vi "Tab as Wizard.vi"() -> ()   [LabVIEW 2014]
panel:
  in  "Next":bool
  in  "stop":bool
  in  "Tab Control":enum32{"Page 1", "Page 2", "Page 3", "Page 4"}(tab)
  # "Page 1"
  # "Page 2"
  # "Page 3"
  # "Page 4"
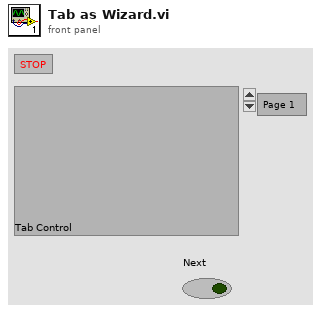
[diagram p1: front panel]
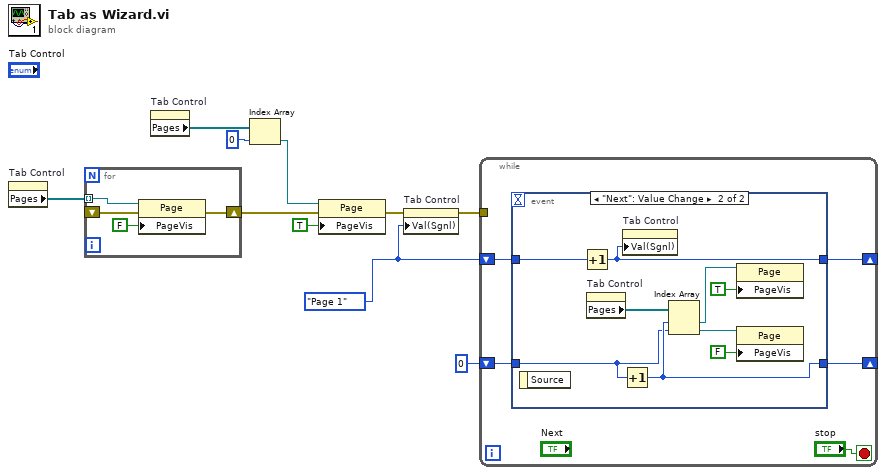
[diagram p0: block diagram]
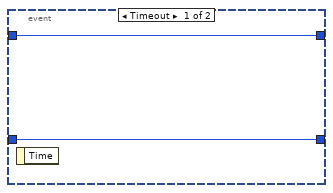
[diagram p2: hidden frame]
diagram:
  w1 = enum32{"Page 1", "Page 2", "Page 3", "Page 4"}."Page 1" ("Tab Control")
  n1 = property on="Tab Control" class="TabCtl (strict)"() -> ("Pages"=w8:refnum<vi>[])  [unwired: 2 in, 2 out]
  n2 = for {
    tunnel: w8 -> [w14] mode=indexing
    shift-right: [w12] -> w4
    shift-left: _ -> [w11]
    n3 = property class="Page"(reference=w14, error in=w11, "PageVis"=FALSE ("Page Visible")) -> (error out=w12:errorcluster)  [unwired: 1 out]
  }
  n4 = property on="Tab Control" class="TabCtl (strict)"() -> ("Pages"=w7:refnum<vi>[])  [unwired: 2 in, 2 out]
  n5 = Index Array(array=w7, index=0) -> (element=w5:refnum<vi>)
  n6 = property class="Page"(reference=w5, error in=w4, "PageVis"=TRUE ("Page Visible")) -> (error out=w2:errorcluster)  [unwired: 1 out]
  n7 = property on="Tab Control" class="TabCtl (strict)"(error in=w2, "Val(Sgnl)"=w1) -> (error out=w10:errorcluster)  [unwired: 1 in, 1 out]
  n8 = while {
    tunnel: w10 -> [_]
    shift-right: [w17] -> _
    shift-left: w1 -> [w18]
    shift-right: [w15] -> _
    shift-left: u16 0 -> [w16]
    stop <- "stop" stop-if-true
    n9 = event shown="[1] \"Next\": Value Change" {
      selector: _ -> [_ _]
      dyn-events: _ -> [_ _]
      timeout: _ -> [_ _]
      tunnel: w18 -> [w20 w30]
      tunnel: [w20 w29] -> w17
      tunnel: w16 -> [w21 w24]
      tunnel: [w21 w27] -> w15
      event Timeout {
        n10 = event-data() -> ()  [unwired: 1 in, 1 out]
      }
      event "Next": Value Change {
        n11 = event-data() -> ()  [unwired: 1 in, 1 out]
        n12 = Increment(x=w30) -> (x+1=w29:enum32{"Page 1", "Page 2", "Page 3", "Page 4"})
        n13 = property on="Tab Control" class="TabCtl (strict)"() -> ("Pages"=w28:refnum<vi>[])  [unwired: 2 in, 2 out]
        n14 = Increment(x=w24) -> (x+1=w27:u16)
        n15 = property on="Tab Control" class="TabCtl (strict)"("Val(Sgnl)"=w29) -> ()  [unwired: 2 in, 2 out]
        n16 = Index Array(array=w28, index #1=w27, index #2=w24) -> (element #1=w26:refnum<vi>, element #2=w23:refnum<vi>)
        n17 = property class="Page"(reference=w26, "PageVis"=TRUE ("Page Visible")) -> ()  [unwired: 1 in, 2 out]
        n18 = property class="Page"(reference=w23, "PageVis"=FALSE ("Page Visible")) -> ()  [unwired: 1 in, 2 out]
      }
    }
  }
